vi "niRFSTS Sequence Flow Create RF Cal Sweep Settings.vi"(0 "Session Handle in":T1, 11 "error in (no error)":errorcluster) -> (4 "Session Handle out":T1, 15 "error out":errorcluster)   [LabVIEW 2016]
uses:
  niRFSTS Sequence Flow.lvclass
  C:/Sequence Automation/Plugins/Sequence Automation Session.lvlibp/Sequence Automation Session.lvclass
  Plugins/QPA Measurement.lvlibp/QPA Measurement.lvclass
  C:/Sequence Automation/Plugins/Measurement Interface.lvlibp/Measurement Interface.lvclass
  C:/Sequence Automation/Plugins/FPF.lvlibp/Factory Plugin Framework.lvclass
  Plugins/String Database.lvlibp/String Database.lvclass
  Typedefs/Session Handle.ctl
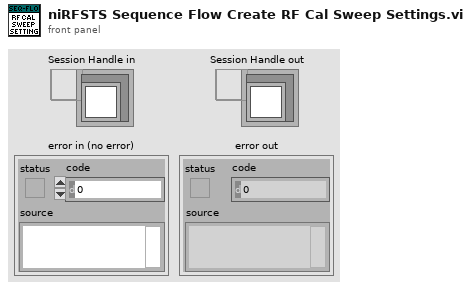
[diagram p1: front panel]
types:
  T1 = typedef "niRFSTS Sequence Flow.lvclass/Session Handle.ctl" = refnum<data-value>
  T2 = typedef "niRFSTS Sequence Flow.lvclass/RF Calibration Parameters.ctl" = cluster{"Test Parameter":string, "SA Pin":string, "SG Pin":string, "Frequency (Hz)":dbl, "Modulation Waveform Alias":string, "Waveform Headroom (dB)":dbl, "RF Power (Step, Servo, List)":string, "Expected Gain (dB)":dbl, "Gain Accuracy (dB)":dbl}
  T3 = typedef "RFPM CLB Calibration UI.lvclass/Sweep Editor Data.ctl" = cluster{"Sweep Name":string, "Sweep Type":T4, "Pin(s)":string, "Sweep Text":string, "Sweep Points":T5[]}
  T4 = typedef "RFPM CLB Calibration UI.lvlibp/RFPM CLB Calibration Process.lvlib/RFPM CLB Calibration Process.lvclass/Sweep Type.ctl" = enum16{"Vector", "Source", "Receiver"}
  T5 = typedef "RFPM CLB Calibration UI.lvclass/Sweep Points.ctl" = cluster{"Frequency":dbl, "Port Power":dbl, "Reference Level":dbl, "TX Path":string, "RX Path":string, "IFBW":dbl}
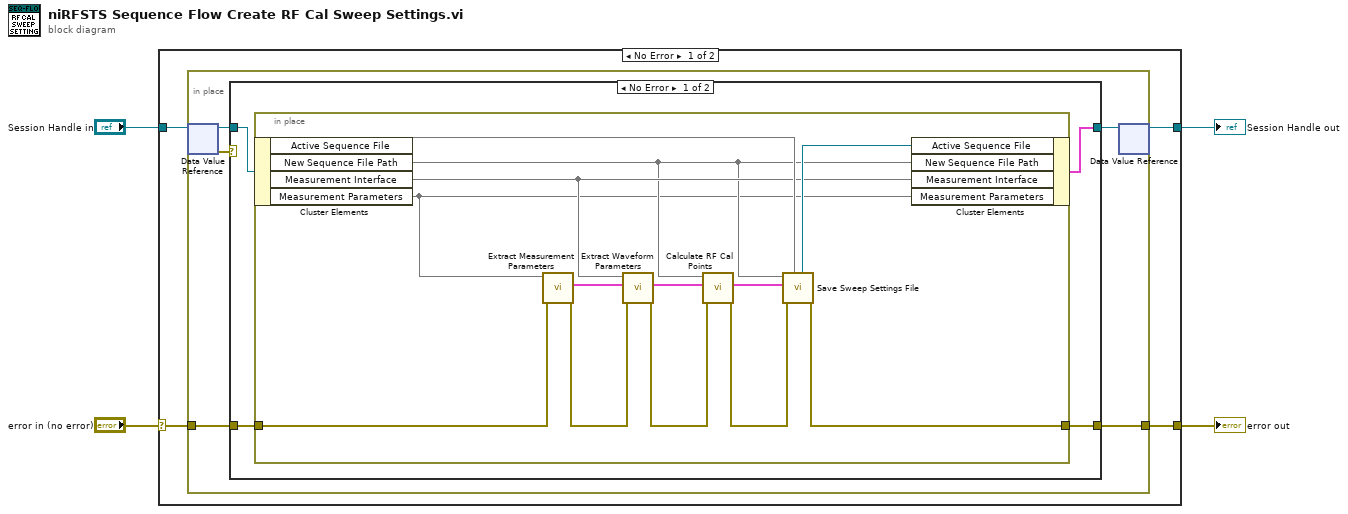
[diagram p0: block diagram]
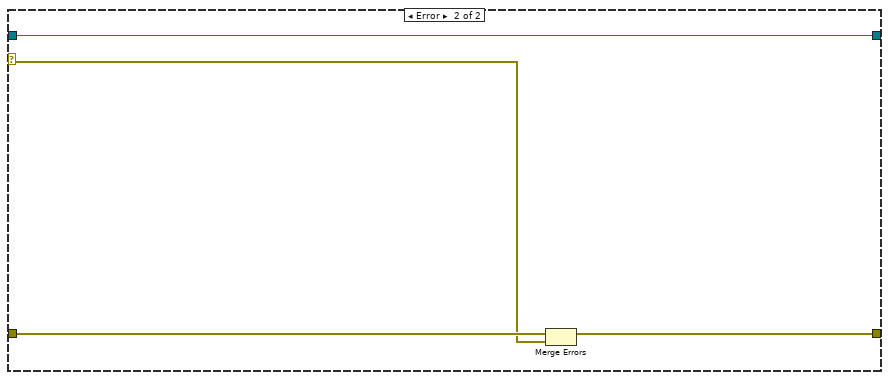
[diagram p2: hidden frame]
diagram:
  n1 = case shown="No Error" "error in (no error)" {
    selector: "error in (no error)" -> [w6 w35]
    tunnel: "Session Handle in" -> [w8 w36]
    tunnel: [w7 w36] -> w3
    tunnel: [w5 w35] -> w2
    frame No Error {
      n2 = in-place {
        in-place-border: w6 -> [w9]
        in-place-border: [w12] -> w5
        n3 = in-place-dvr #1(w8) -> (w13:refnum<class "niRFSTS Sequence Flow.lvclass">, w10:errorcluster)
        n4 = case shown="No Error" w10 {
          selector: w10 -> [_ w33]
          tunnel: w13 -> [w15 w31]
          tunnel: [w16 w32] -> w12
          tunnel: [w14 w31] -> w11
          tunnel: w9 -> [w17 w34]
          frame No Error {
            n5 = in-place {
              in-place-border: w17 -> [w30]
              in-place-border: [w29] -> w16
              n6 = in-place-cluster #2(w15) -> ("Active Sequence File"=w28, "New Sequence File Path"=w25, "Measurement Interface"=w26, "Measurement Parameters"=w24)
              n7 = call "Extract Measurement Parameters.vi"("error in (no error)"=w30, "Measurement Parameters"=w24) -> ("error out"=w23:errorcluster, "RF Calibration Parameters"=w22:T2[])  [unwired: 8 in]
              n8 = call "Extract Waveform Parameters.vi"("error in (no error)"=w23, "RF Calibration Parameters In"=w22, "Measurement Interface"=w26) -> ("error out"=w20:errorcluster, "RF Calibration Parameters Out"=w21:T2[])  [unwired: 7 in]
              n9 = call "Calculate RF Cal Points.vi"("error in (no error)"=w20, "RF Calibration Parameters In"=w21, "New Sequence File Path"=w25) -> ("error out"=w19:errorcluster, "Sweep Settings Data"=w18:T3[])  [unwired: 7 in]
              n10 = call "Save Sweep Settings File.vi"("Seq File Ref In"=w28, "error in (no error)"=w19, "Sweep Settings Data"=w18, "New Sequence File Path"=w25) -> ("error out"=w29:errorcluster, "Seq File Ref Out"=w27:refnum<k7>)  [unwired: 6 in]
              n11 = in-place-cluster #2("Active Sequence File"=w27, "New Sequence File Path"=w25, "Measurement Interface"=w26, "Measurement Parameters"=w24) -> (w14:cluster{})
            }
          }
          frame Error {
            n12 = Merge Errors(w34, w33) -> (w32:errorcluster)
          }
        }
        n13 = in-place-dvr #1(w11) -> (w7:T1)  [unwired: 1 out]
      }
    }
    frame Error {
    }
  }
  "Session Handle out" <- w3
  "error out" <- w2
